vi "Test Configure.vi"(0 "Template Tx Test in":refnum<class "Template RF Test.lvclass">, 11 "error in (no error)":errorcluster) -> (4 "Template Tx Test out":refnum<class "Template RF Test.lvclass">, 15 "error out":errorcluster)   [LabVIEW 2015, in "niDTS Template.lvlib" / "Template RF Test.lvclass"]
uses:
  Template RF Test.lvclass
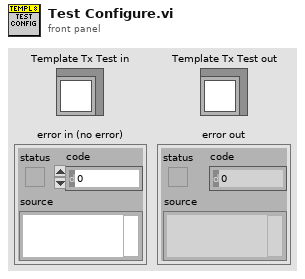
[diagram p1: front panel]
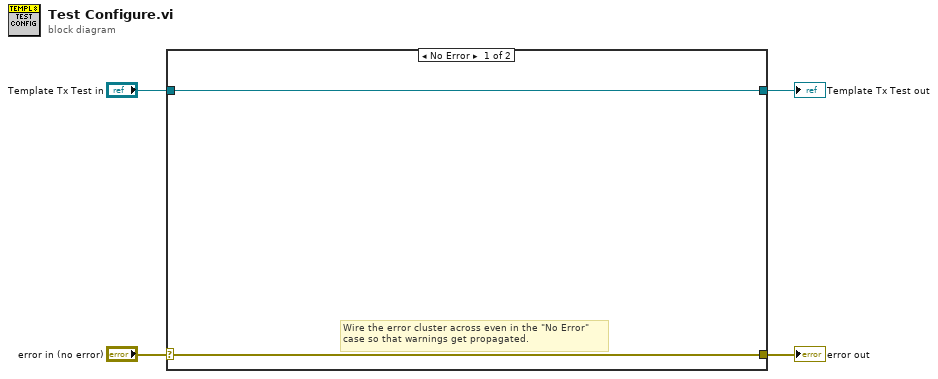
[diagram p0: block diagram]
diagram:
  n1 = case shown="No Error" "error in (no error)" {
    selector: "error in (no error)" -> [w5 w8]
    tunnel: [w5 w8] -> w2
    tunnel: [w6 w7] -> w3
    tunnel: "Template Tx Test in" -> [w6 w7]
    frame No Error {
      # "Wire the error cluster across even in the \"No Error\"\ncase so that warnings get propagated."
    }
    frame Error {
    }
  }
  "error out" <- w2
  "Template Tx Test out" <- w3
